vi "Specify BLM Encoder Resolution.vi"() -> ()   [LabVIEW 2021]
doc: "This VI saves selected encoder resolution of 8000 or 10000 into register #1 of the controller non-volatile memory. It also allows to read the value stored in the register #1 of the controller non-volatile memory.\nUser-defined register #1 is used to pass data beyween the computer and the controller non-volatile memory."
panel:
  in  "Error In":errorcluster
  out "Encoder Resolution":dbl
  in  "Write Resolution":bool
  in  "Read Resolution":bool
  in  "Test Connection":bool
  out "Test Results":string
  out "Error Out":errorcluster {"code" format="%.0x"}
  in  "stop":bool
  in  "MOTOR (BLM) Address":refnum<visa-resource-name>
  # "READ ME FIRST\nUsed non-volatile memory is limited to\napproximately 10,000 write cycles. \nDo not use WRITE operation without needs.\n\nValue  in the Encoder Resolution window blinks to confirm successful reading operation.\n\n1. Select The Motor (BLM) address\n2. Run this VI\n3. Click \"Test connection\" button\n4. Click \"READ encoder resolution\" button\n    If the \"Encoder Resolution\" window shows 8000 or 10000, the controller is already configured properly. Go to step 8. \n    Overwise Go to step 5. \n5. Click  \"WRITE encoder resolution\" button\n6. Click  the appropriate  encoder resolution in the appeared window\n7. A dialog window will notify you on the result.\n8. Stop and close this VI.  BLM_ManualControl.vi should work properly."
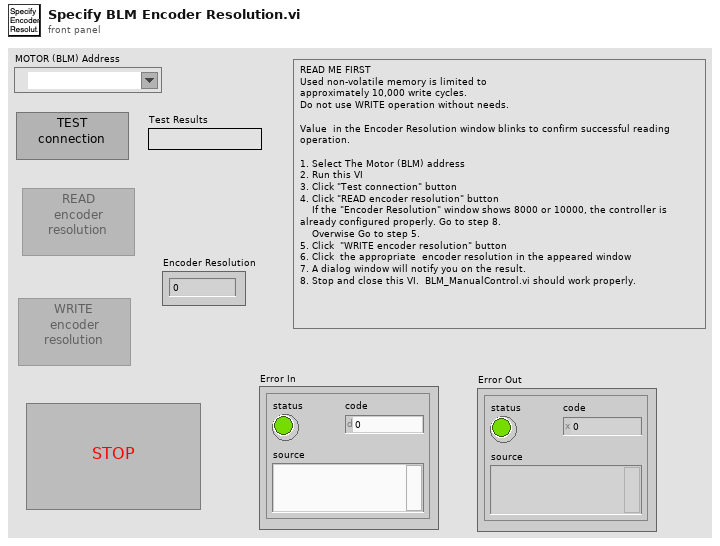
[diagram p1: front panel]
types:
  T1 = enum8{"Enabled", "Disabled", "Disabled and Grayed Out"}
  T2 = enum16{"Left Button", "Center Button", "Right Button", "Window Close"}
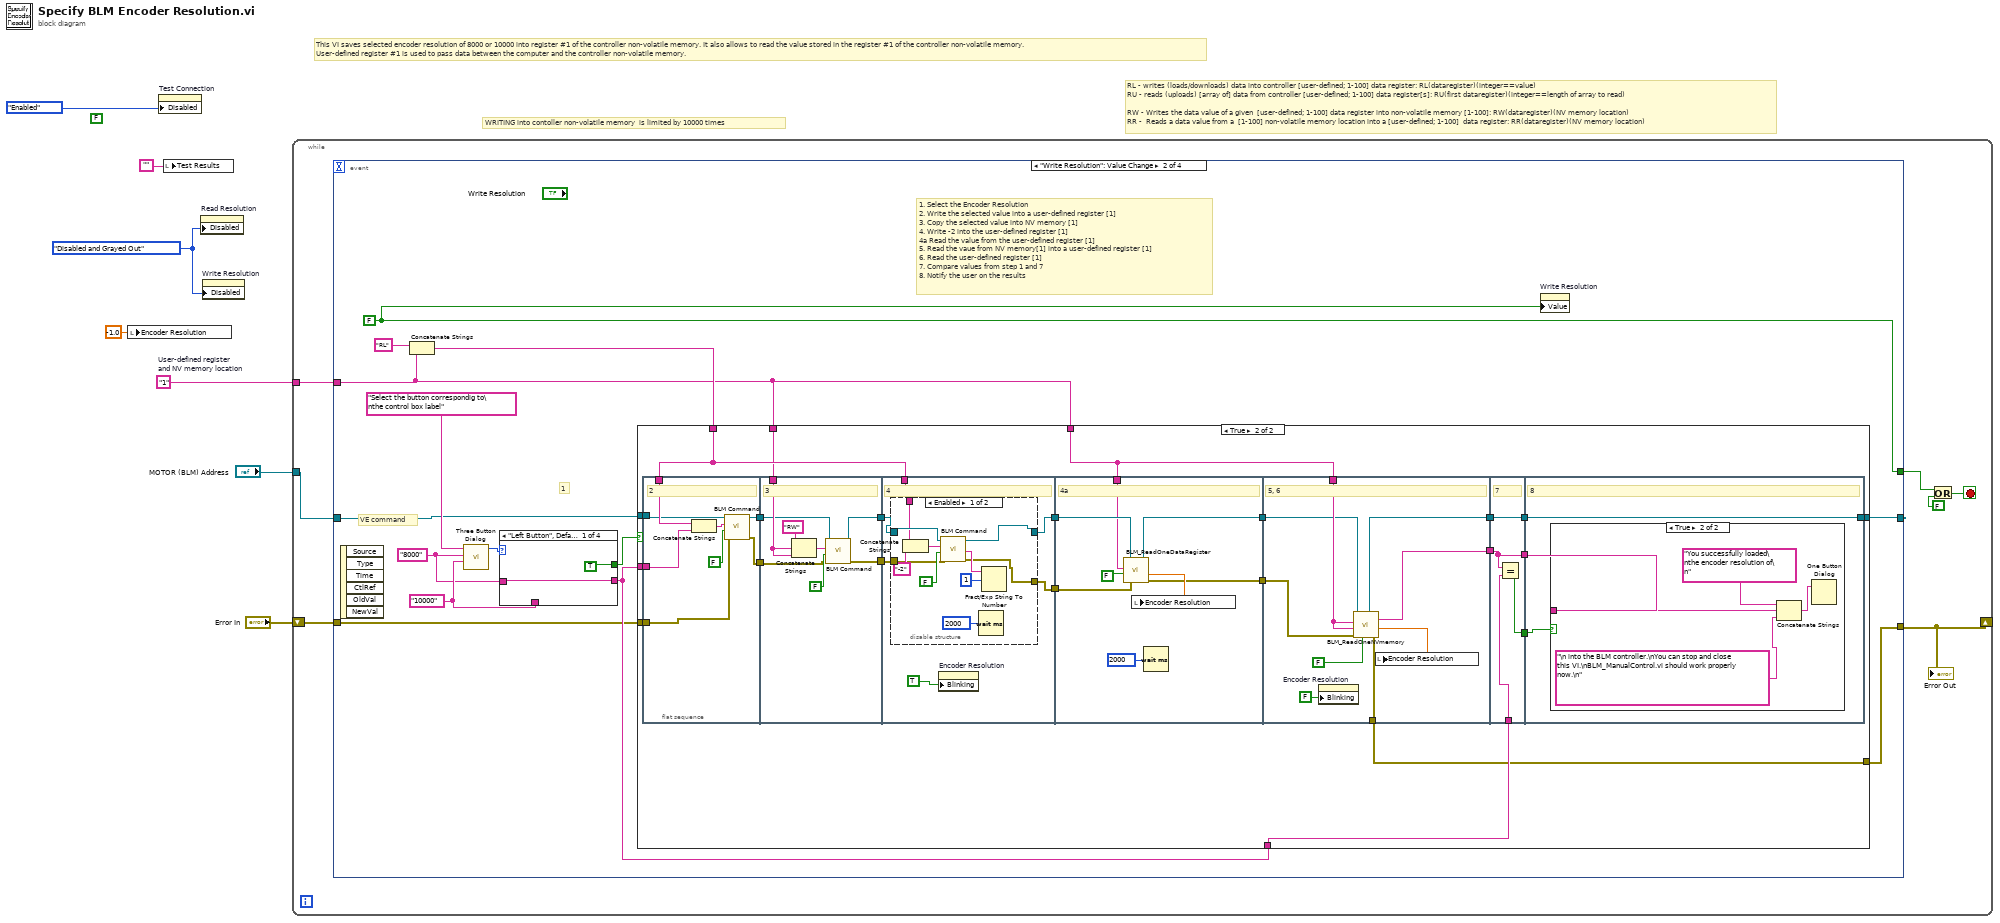
[diagram p0: block diagram]
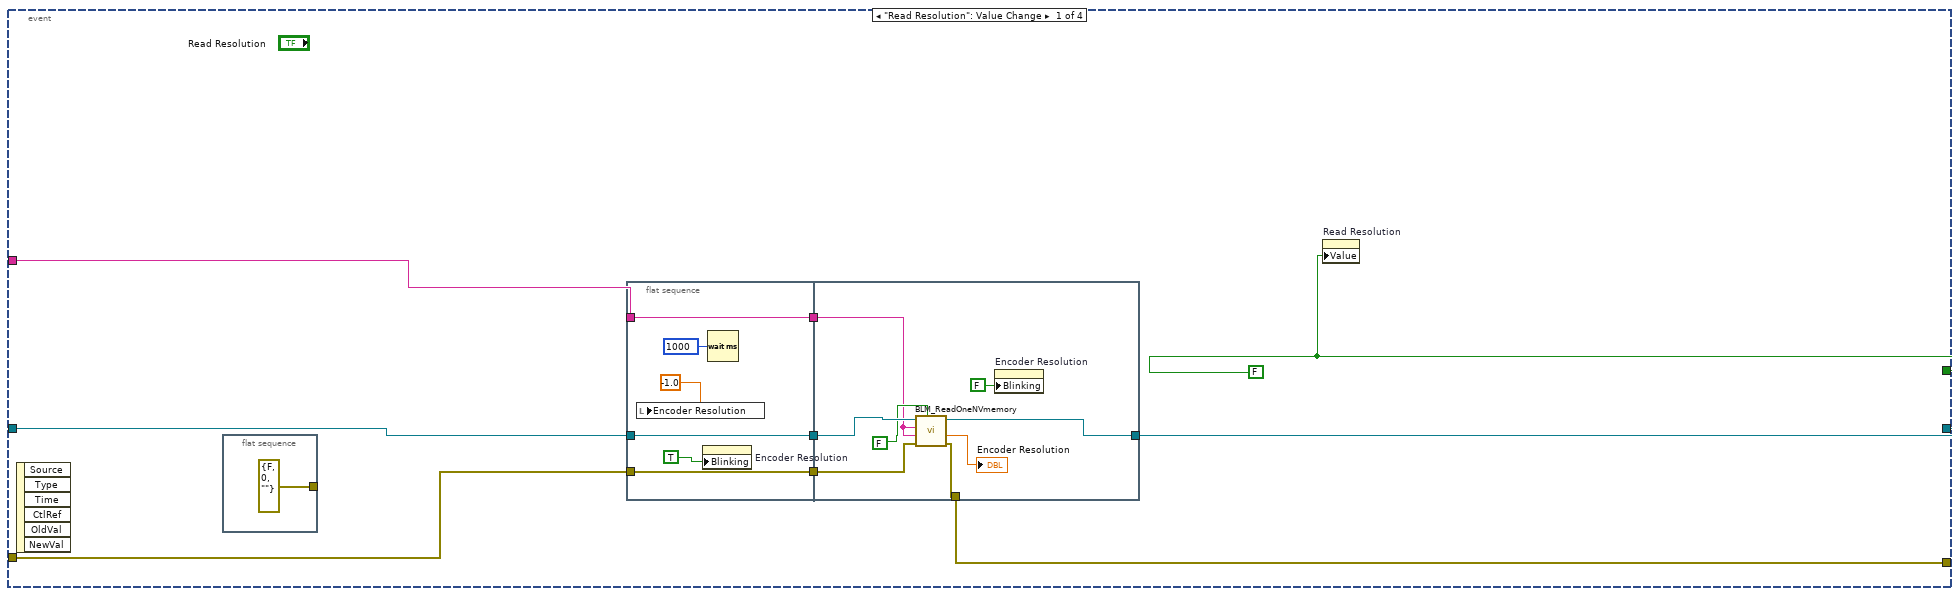
[diagram p2: hidden frame]
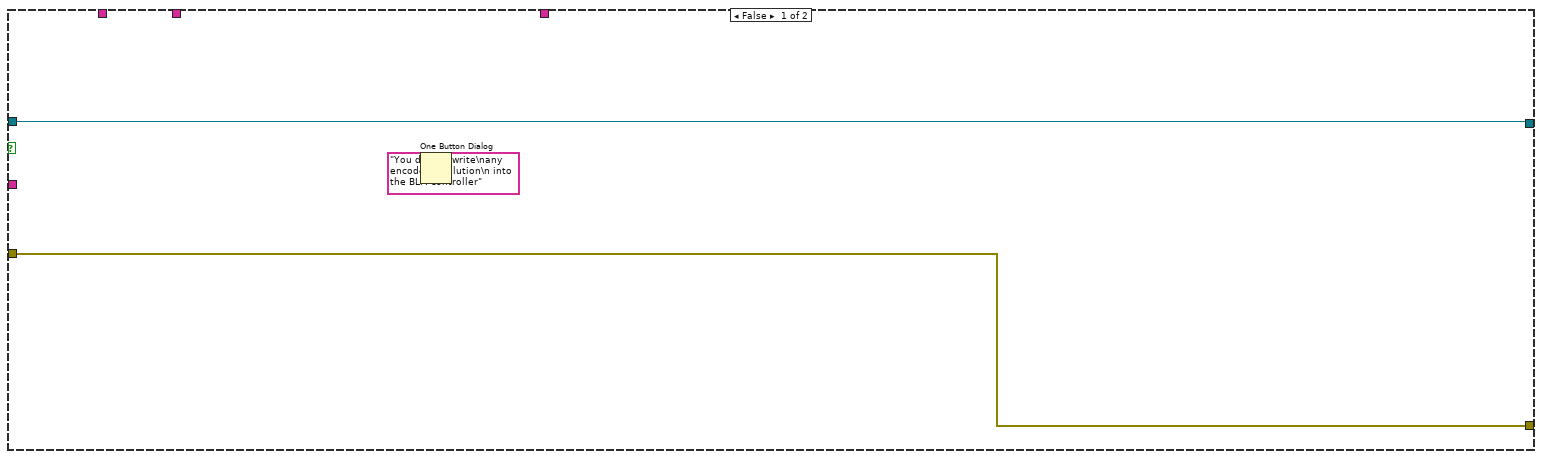
[diagram p3: hidden frame]
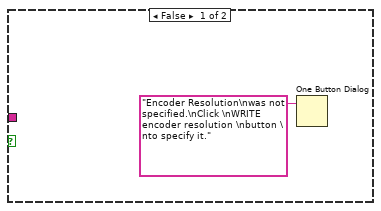
[diagram p5: hidden frame]
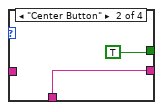
[diagram p6: hidden frame]
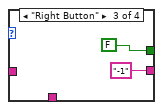
[diagram p7: hidden frame]
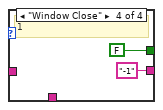
[diagram p8: hidden frame]
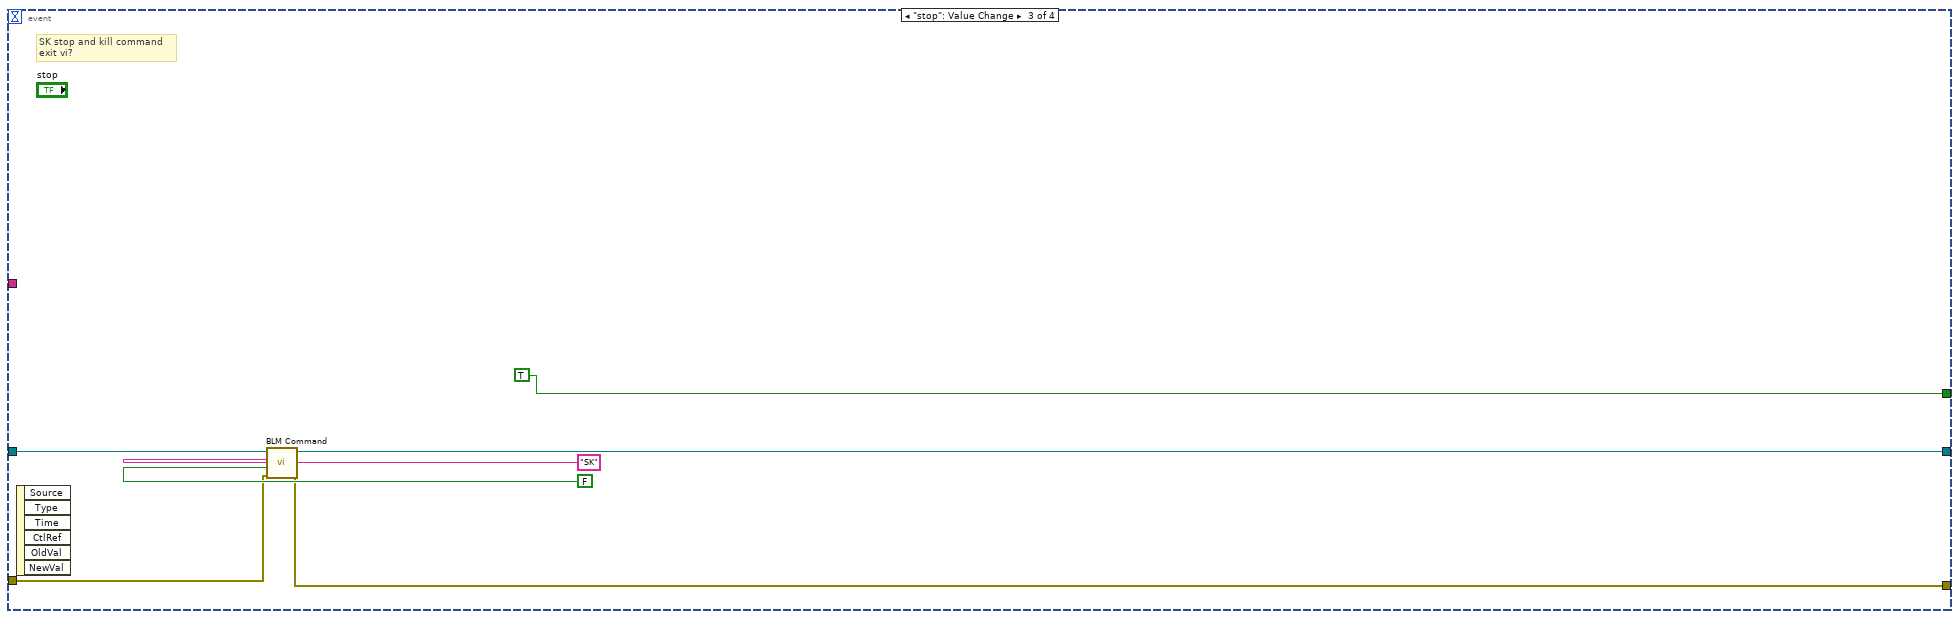
[diagram p9: hidden frame]
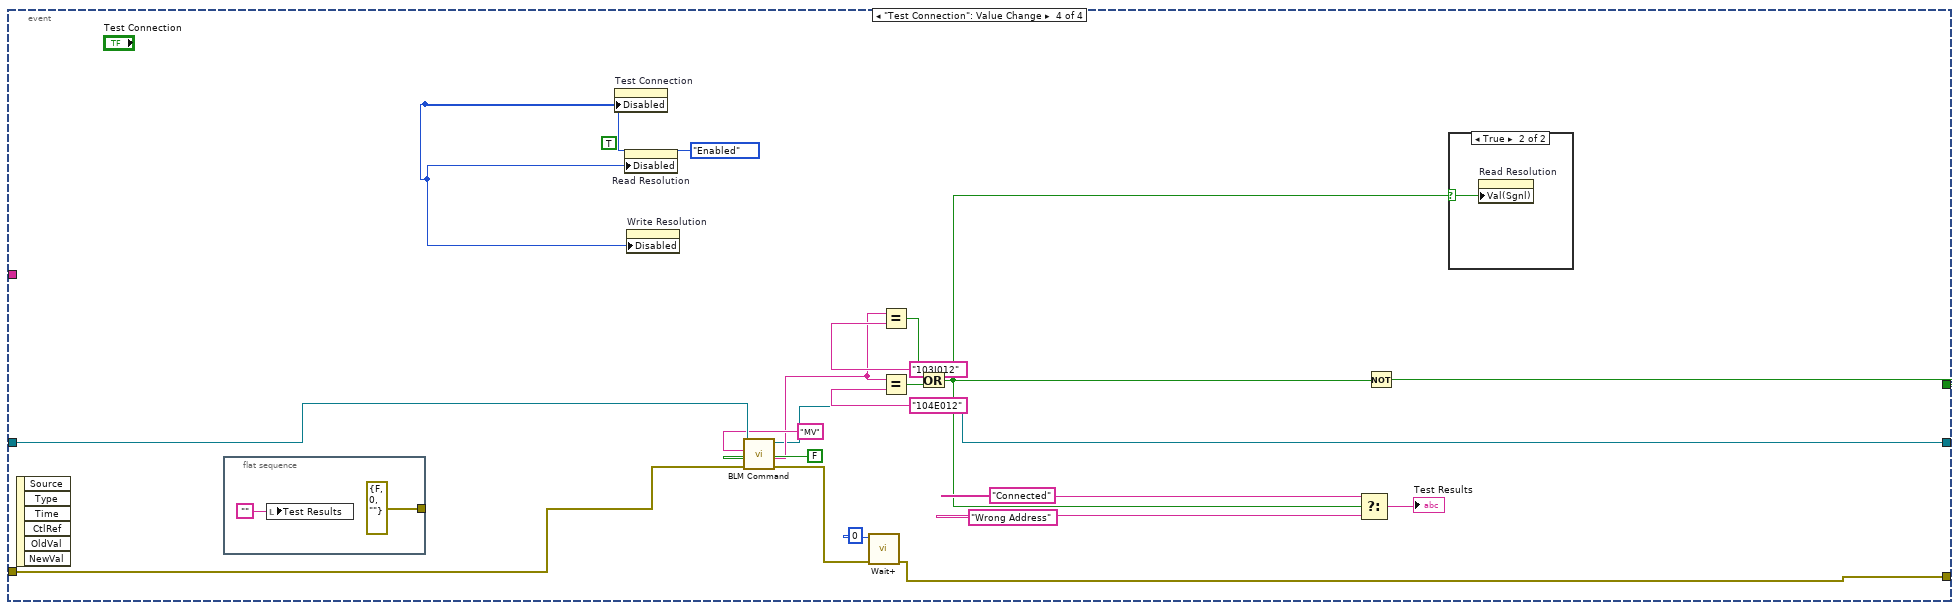
[diagram p10: hidden frame]
diagram:
  w2 = "1"  # User-defined register and NV memory location
  (unwired) FALSE ("Read Echo?")
  w4 = T1."Disabled and Grayed Out" ("Disabled")
  # "This VI saves selected encoder resolution of 8000 or 10000 into register #1 of the controller non-volatile memory. It also allows to read the value stored in the register #1 of the controller non-volatile memory.\nUser-defined register #1 is used to pass data between the computer and the controller non-volatile memory."
  # "WRITING into contoller non-volatile memory  is limited by 10000 times"
  # "RL - writes (loads/downloads) data into controller [user-defined; 1-100] data register: RL(dataregister)(integer==value)\nRU - reads (uploads) [array of] data from controller [user-defined; 1-100] data register[s]: RU(first dataregister)(integer==length of array to read)\n\nRW - Writes the data value of a given  [user-defined; 1-100] data register into non-volatile memory [1-100]: RW(dataregister)(NV memory location)\nRR -  Reads a data value from a  [1-100] non-volatile memory location into a [user-defined; 1-100]  data register: RR(dataregister)(NV memory location)"
  n1 = local write "Encoder Resolution"(-1.0 ("Encoder Resolution")) -> ()
  n2 = property on="Test Connection" class="Bool"("Disabled"=T1."Enabled") -> ()  [unwired: 2 in, 2 out]
  n3 = local write "Test Results"("" ("Response")) -> ()
  n4 = property on="Read Resolution" class="Bool (strict)"("Disabled"=w4) -> ()  [unwired: 2 in, 2 out]
  n5 = property on="Write Resolution" class="Bool (strict)"("Disabled"=w4) -> ()  [unwired: 2 in, 2 out]
  n6 = while {
    tunnel: "MOTOR (BLM) Address" -> [w14]
    tunnel: w2 -> [w11]
    shift-right: [w9] -> _
    shift-left: "Error In" -> [w10]
    stop <- w12 stop-if-true
    n7 = event shown="[1] \"Write Resolution\": Value Change" {
      selector: _ -> [_ _ _ _]
      dyn-events: _ -> [_ _ _ _]
      timeout: _ -> [_ _ _ _]
      tunnel: w14 -> [w22 w47 w155 w174]
      tunnel: [w21 w52 TRUE w172] -> w13
      tunnel: [w23 w51 w151 w160] -> _
      tunnel: w11 -> [w18 w41 _ _]
      tunnel: w10 -> [w16 w40 w150 w156]
      tunnel: [w15 w39 w149 w157] -> w9
      event "Read Resolution": Value Change {
        w21 = FALSE
        n8 = event-data() -> ()  [unwired: 1 in, 6 out]
        n9 = flat-sequence {
          tunnel: [errorcluster {"status"=FALSE, "code"=0, "source"=""} ("error in (no error)")] -> _
          frame #0 {
          }
        }
        n10 = flat-sequence {
          tunnel: w16 -> [w28]
          tunnel: w22 -> [w29]
          tunnel: [w29] -> w20
          tunnel: [w28] -> w19
          tunnel: w18 -> [w25]
          tunnel: [w25] -> w17
          tunnel: [w30] -> w23
          tunnel: w20 -> [w35]
          tunnel: w19 -> [w33]
          tunnel: w17 -> [w32]
          tunnel: [w31] -> w15
          frame #0 {
            n11 = local write "Encoder Resolution"(-1.0 ("Encoder Resolution")) -> ()
            n12 = property on="Encoder Resolution" class="DigNum (strict)"("Blinking"=TRUE) -> ()  [unwired: 2 in, 2 out]
            n13 = Wait (ms)(milliseconds to wait=u32 1000) -> ()  [unwired: 1 out]
          }
          frame #1 {
            n14 = call "BLM_ReadOneNVmemory.vi"("Read Echo?"=FALSE, "error in (no error)"=w33, "Transit \nuser-defined register#"=w32, "NV memory #"=w32, "Port Address"=w35) -> ("error out"=w31:errorcluster, "NV memory value"=→"Encoder Resolution":dbl, "Port Address Out"=w30:refnum<visa-resource-name>)  [unwired: 1 out]
            n15 = property on="Encoder Resolution" class="DigNum (strict)"("Blinking"=FALSE) -> ()  [unwired: 2 in, 2 out]
          }
        }
        n16 = property on="Read Resolution" class="Bool (strict)"("Value"=w21) -> ()  [unwired: 2 in, 2 out]
      }
      event "Write Resolution": Value Change {
        w46 = "10000" ("Center Button Text (\"No\")")
        w45 = "8000" ("Left Button Text (\"Yes\")")
        w52 = FALSE
        # "1"
        # "1. Select the Encoder Resolution\n2. Write the selected value into a user-defined register [1]\n3. Copy the selected value into NV memory [1]\n4. Write -2 into the user-defined register [1]\n4a Read the value from the user-defined register [1]\n5. Read the vaue from NV memory[1] into a user-defined register [1]\n6. Read the user-defined register [1]\n7. Compare values from step 1 and 7\n8. Notify the user on the results"
        # "VE command"
        n17 = event-data() -> ()  [unwired: 1 in, 6 out]
        n18 = Concatenate Strings("RL" ("string (\"\")"), w41) -> (w43:string)
        n19 = call <vilib>:"Three Button Dialog.vi"("Center Button Text (\"No\")"=w46, "Left Button Text (\"Yes\")"=w45, "message"="Select the button correspondig to\nthe control box label") -> ("Which Button?"=w49:T2)  [unwired: 8 in]
        n20 = case shown="\"Left Button\", Default" w49 {
          tunnel: w46 -> [_ w144 _ _]
          tunnel: [w142 w144 "-1" ("Center Button Text (\"No\")") "-1" ("Center Button Text (\"No\")")] -> w42
          tunnel: w45 -> [w142 _ _ _]
          tunnel: [TRUE TRUE FALSE FALSE] -> w44
          frame "Left Button", Default {
          }
          frame "Center Button" {
          }
          frame "Right Button" {
          }
          frame "Window Close" {
            # "1"
          }
        }
        n21 = case shown="True" w44 {
          tunnel: [w55 w77] -> w51
          tunnel: w43 -> [_ w70]
          tunnel: w47 -> [w55 w76]
          tunnel: w42 -> [_ w75]
          tunnel: w42 -> [_ w71]
          tunnel: w41 -> [_ w68]
          tunnel: w41 -> [_ w63]
          tunnel: w40 -> [w53 w57]
          tunnel: [w53 w56] -> w39
          frame False {
            n22 = One Button Dialog(message="You did not write\nany encoder resolution\n into the BLM controller") -> ()  [unwired: 1 in, 1 out]
          }
          frame True {
            n23 = flat-sequence {
              tunnel: w70 -> [w82]
              tunnel: w76 -> [w81]
              tunnel: w75 -> [w80]
              tunnel: [w84] -> w74
              tunnel: [w79] -> w58
              tunnel: w57 -> [w78]
              tunnel: w74 -> [w88]
              tunnel: w63 -> [w90]
              tunnel: [w89] -> w62
              tunnel: [w87] -> w61
              tunnel: w58 -> [w86]
              tunnel: w70 -> [w97]
              tunnel: [w99] -> w69
              tunnel: w62 -> [w98]
              tunnel: w61 -> [w95]
              tunnel: [w94] -> w60
              tunnel: w69 -> [w118]
              tunnel: w68 -> [w117]
              tunnel: [w115] -> w67
              tunnel: w60 -> [w113]
              tunnel: [w112] -> w59
              tunnel: [w125] -> w73
              tunnel: w68 -> [w127]
              tunnel: w67 -> [w124]
              tunnel: [w123] -> w66
              tunnel: w59 -> [w121]
              tunnel: [w120] -> w56
              tunnel: w73 -> [w132]
              tunnel: [w132] -> w72
              tunnel: w71 -> [w131]
              tunnel: w66 -> [w130]
              tunnel: [w130] -> w65
              tunnel: [w129] -> w64
              tunnel: [w135] -> w77
              tunnel: w72 -> [w135]
              tunnel: w65 -> [w134]
              tunnel: w64 -> [w133]
              frame #0 {
                # "2"
                n24 = Concatenate Strings(w82, w80) -> (w83:string)
                n25 = call "BLM Command.vi"("error in (no error)"=w78, "Read Echo?"=FALSE, "Command"=w83, "Port Address"=w81) -> ("error out"=w79:errorcluster, "Port Address Out"=w84:refnum<visa-resource-name>)  [unwired: 2 in, 3 out]
              }
              frame #1 {
                # "3"
                n26 = Concatenate Strings("RW" ("string"), w90, w90) -> (w92:string)
                n27 = call "BLM Command.vi"("error in (no error)"=w86, "Read Echo?"=FALSE, "Command"=w92, "Port Address"=w88) -> ("error out"=w87:errorcluster, "Port Address Out"=w89:refnum<visa-resource-name>)  [unwired: 2 in, 3 out]
              }
              frame #2 {
                # "4"
                n28 = disable-structure shown="Enabled" {
                  disable-tunnel: [w106 w111] -> w99
                  disable-tunnel: w98 -> [w105 w111]
                  disable-tunnel: w97 -> [w104 _]
                  disable-tunnel: w95 -> [w101 _]
                  disable-tunnel: [w100 _] -> w94
                  frame Enabled {
                    n29 = Concatenate Strings(w104, "-2" ("string")) -> (w108:string)
                    n30 = call "BLM Command.vi"("error in (no error)"=w101, "Read Echo?"=FALSE, "Command"=w108, "Port Address"=w105) -> ("error out"=w100:errorcluster, "Response"=w107:string, "Port Address Out"=w106:refnum<visa-resource-name>)  [unwired: 2 in, 2 out]
                    n31 = Wait (ms)(milliseconds to wait=u32 2000) -> ()  [unwired: 1 out]
                    n32 = Fract/Exp String To Number(string=w107, offset=1) -> ()  [unwired: 2 in, 2 out]
                  }
                  frame Disabled {
                  }
                }
                n33 = property on="Encoder Resolution" class="DigNum (strict)"("Blinking"=TRUE) -> ()  [unwired: 2 in, 2 out]
              }
              frame #3 {
                # "4a"
                n34 = call "BLM_ReadOneDataRegister.vi"("error in (no error)"=w113, "Read Echo?"=FALSE, "Register#"=w117, "Port Address"=w118) -> ("error out"=w112:errorcluster, "Register Value"=w116:dbl, "Port Address Out"=w115:refnum<visa-resource-name>)  [unwired: 1 out]
                n35 = local write "Encoder Resolution"(w116) -> ()
                n36 = Wait (ms)(milliseconds to wait=u32 2000) -> ()  [unwired: 1 out]
              }
              frame #4 {
                # "5, 6"
                n37 = property on="Encoder Resolution" class="DigNum (strict)"("Blinking"=FALSE) -> ()  [unwired: 2 in, 2 out]
                n38 = call "BLM_ReadOneNVmemory.vi"("Read Echo?"=FALSE, "error in (no error)"=w121, "Transit \nuser-defined register#"=w127, "NV memory #"=w127, "Port Address"=w124) -> ("error out"=w120:errorcluster, "NV memory value"=w126:dbl, "NV memory string"=w123:string, "Port Address Out"=w125:refnum<visa-resource-name>)
                n39 = local write "Encoder Resolution"(w126) -> ()
              }
              frame #5 {
                # "7"
                n40 = Equal?(x=w130, y=w131) -> (x = y?=w129:bool)
              }
              frame #6 {
                # "8"
                n41 = case shown="True" w133 {
                  tunnel: w134 -> [_ w137]
                  frame False {
                    n42 = One Button Dialog(message="Encoder Resolution\nwas not specified.\nClick \nWRITE encoder resolution \nbutton \nto specify it.") -> ()  [unwired: 1 in, 1 out]
                  }
                  frame True {
                    n43 = Concatenate Strings("You successfully loaded\nthe encoder resolution of\n" ("message"), w137, "\n into the BLM controller.\nYou can stop and close this VI.\nBLM_ManualControl.vi should work properly now.\n" ("string")) -> (w139:string)
                    n44 = One Button Dialog(message=w139) -> ()  [unwired: 1 in, 1 out]
                  }
                }
              }
            }
          }
        }
        n45 = property on="Write Resolution" class="Bool (strict)"("Value"=w52) -> ()  [unwired: 2 in, 2 out]
      }
      event "stop": Value Change {
        # "SK stop and kill command\nexit vi?"
        n46 = event-data() -> ()  [unwired: 1 in, 6 out]
        n47 = call "BLM Command.vi"("error in (no error)"=w150, "Read Echo?"=FALSE, "Command"="SK", "Port Address"=w155) -> ("error out"=w149:errorcluster, "Port Address Out"=w151:refnum<visa-resource-name>)  [unwired: 2 in, 3 out]
      }
      event "Test Connection": Value Change {
        w159 = T1."Enabled" ("Disabled")
        (unwired) TRUE ("Parameter changed")
        n48 = event-data() -> ()  [unwired: 1 in, 6 out]
        n49 = flat-sequence {
          tunnel: [errorcluster {"status"=FALSE, "code"=0, "source"=""} ("error in (no error)")] -> _
          frame #0 {
            n50 = local write "Test Results"("" ("Response")) -> ()
          }
        }
        n51 = property on="Test Connection" class="Bool"("Disabled"=w159) -> ()  [unwired: 2 in, 2 out]
        n52 = property on="Read Resolution" class="Bool (strict)"("Disabled"=w159) -> ()  [unwired: 2 in, 2 out]
        n53 = property on="Write Resolution" class="Bool (strict)"("Disabled"=w159) -> ()  [unwired: 2 in, 2 out]
        n54 = call "BLM Command.vi"("error in (no error)"=w156, "Read Echo?"=FALSE, "Command"="MV", "Port Address"=w174) -> ("error out"=w171:errorcluster, "Response"=w163:string, "Port Address Out"=w160:refnum<visa-resource-name>)  [unwired: 2 in, 2 out]
        n55 = call "Wait+.vi"("Error In"=w171, "milliseconds to wait"=u32 0) -> ("Error Out"=w157:errorcluster)  [unwired: 4 in, 1 out]
        n56 = Equal?(x=w163, y="103J012" ("Response")) -> (x = y?=w173:bool)
        n57 = Equal?(x=w163, y="104E012" ("Response")) -> (x = y?=w162:bool)
        n58 = Or(x=w173, y=w162) -> (x .or. y?=w158:bool)
        n59 = Select(t="Connected" ("Response"), s=w158, f="Wrong Address" ("Response")) -> (s? t:f=→"Test Results":string)
        n60 = Not(x=w158) -> (.not. x?=w172:bool)
        n61 = case shown="True" w158 {
          selector: w158 -> [_ w175]
          frame False {
          }
          frame True {
            n62 = property on="Read Resolution" class="Bool (strict)"("Val(Sgnl)"=w175) -> ()  [unwired: 2 in, 2 out]
          }
        }
      }
    }
    "Error Out" <- w9
    n63 = Or(x=w13, y=FALSE ("Stop Button")) -> (x .or. y?=w12:bool)
  }
